vi "Shared Variable Client - DataSocket API.vi"() -> ()   [LabVIEW 2016]
doc: "This client VI connects to Shared Variable Server.vi by using the DataSocket API to read the server variable values."
panel:
  out "Monitor Value 2":dbl(knob) scale=0.0..1.0
  out "Monitor Value 1":dbl(knob) scale=0.0..1.0
  in  "Stop":bool
  # "Overview: Demonstrates the use of the DataSocket functions to read shared variable data from a server VI.\nRequirements: Windows\nInstructions:\n1. Make sure Shared Variable Server.vi is already running.\n2. Run this VI. It will read the values of the server shared variables through the DataSocket API.\n3. Click Stop to stop the VI."
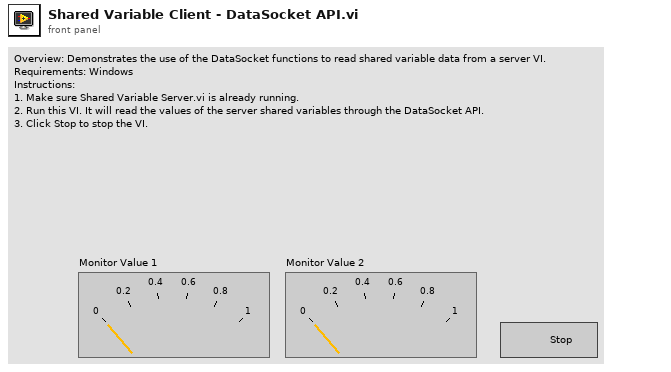
[diagram p1: front panel]
types:
  T1 = enum16{"Read", "Write", "ReadWrite", "BufferedRead", "BufferedReadWrite"}
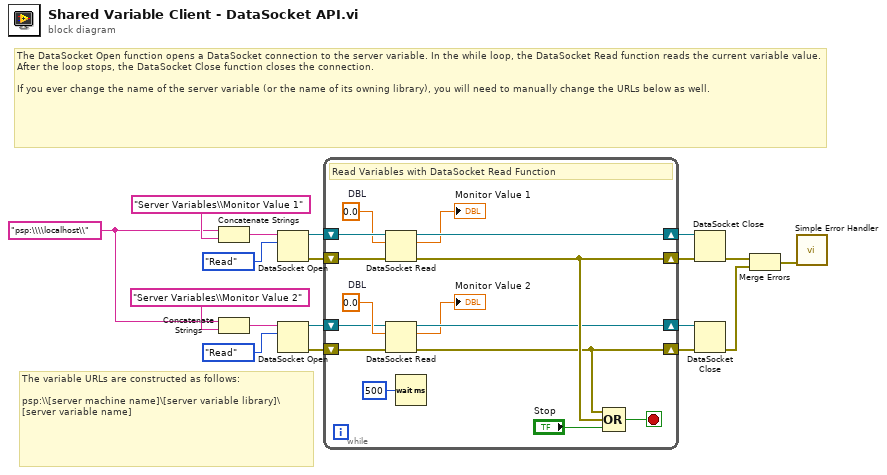
[diagram p0: block diagram]
diagram:
  w1 = "psp:\\\\localhost\\" ("string")
  # "The DataSocket Open function opens a DataSocket connection to the server variable. In the while loop, the DataSocket Read function reads the current variable value. After the loop stops, the DataSocket Close function closes the connection.\n\nIf you ever change the name of the server variable (or the name of its owning library), you will need to manually change the URLs below as well."
  # "The variable URLs are constructed as follows:\n\npsp:\\\\[server machine name]\\[server variable library]\\[server variable name]"
  n1 = Concatenate Strings(w1, "Server Variables\\Monitor Value 1") -> (w17:string)
  n2 = Concatenate Strings(w1, "Server Variables\\Monitor Value 2") -> (w7:string)
  n3 = DataSocket Open(10:T1."Read" ("mode"), 11:w17) -> (0:w13:errorcluster, 3:w12:refnum<k13>)  [unwired: 2 in]
  n4 = DataSocket Open(10:T1."Read" ("mode"), 11:w7) -> (0:w10:errorcluster, 3:w11:refnum<k13>)  [unwired: 2 in]
  n5 = while {
    shift-right: [w32] -> w14
    shift-left: w12 -> [w31]
    shift-right: [w29] -> w16
    shift-left: w13 -> [w30]
    shift-right: [w21] -> w9
    shift-left: w11 -> [w22]
    shift-right: [w19] -> w8
    shift-left: w10 -> [w23]
    stop <- w28 stop-if-true
    w24 = 0.0  # DBL
    w26 = 0.0  # DBL
    # "Read Variables with DataSocket Read Function"
    n6 = DataSocket Read(8:w30, 10:w26, 11:w31) -> (0:w29:errorcluster, 2:→"Monitor Value 1":dbl, 3:w32:refnum<k13>)  [unwired: 2 in, 4 out]
    n7 = DataSocket Read(8:w23, 10:w24, 11:w22) -> (0:w19:errorcluster, 2:→"Monitor Value 2":dbl, 3:w21:refnum<k13>)  [unwired: 2 in, 4 out]
    n8 = Wait (ms)(milliseconds to wait=u32 500 ("millisecond multiple")) -> ()  [unwired: 1 out]
    n9 = Compound Arithmetic op=OR(w19, w29, "Stop") -> (w28:bool)
  }
  n10 = DataSocket Close(8:w16, 11:w14) -> (0:w15:errorcluster)  [unwired: 1 in, 1 out]
  n11 = DataSocket Close(8:w8, 11:w9) -> (0:w3:errorcluster)  [unwired: 1 in, 1 out]
  n12 = Merge Errors(w15, w3) -> (w4:errorcluster)
  n13 = call <vilib>:"Simple Error Handler.vi"("error in (no error)"=w4) -> ()  [unwired: 4 in, 5 out]
